vi "Calibrate.vi"(6 "Uncertainty (%) Vin":dbl=1.0, 7 "V_in (V)":dbl=5.0, 8 "Uncertainty (%) Resistor":dbl=1.0, 9 "Resistor (ohms)":dbl=10000.0, 10 "Uncertainty (%) Temp":dbl=1.0, 11 "Temperature (K)":dbl=292.15) -> (0 "Calib Temperature":dbl=292.15, 1 "Uncertainty Calib Temp":dbl=1.0, 2 "Uncertainty (%) Thermistor":dbl=2.9457081958270703, 3 "Calibration Resistance (ohms)":dbl=8620.698071334564, 4 "Canceled":bool, 5 "error out":errorcluster)   [LabVIEW 2013]
panel:
  out "V_out (V)":dbl=2.3148160284617916
  in  "Stop Button":bool
  in  "Calibrate":bool
  in  "Set V_in":bool
  in  "Set V_out":bool
  in  "Set Resistor":bool
  in  "Uncertainty (%) Vout":dbl=1.0
  # "NOTE:\nDO NOT PLAY WITH THIS UNLESS YOU KNOW\nWHAT YOU ARE DOING.\nIncorrect calibration may lead to hardware damage!"
  # "Options"
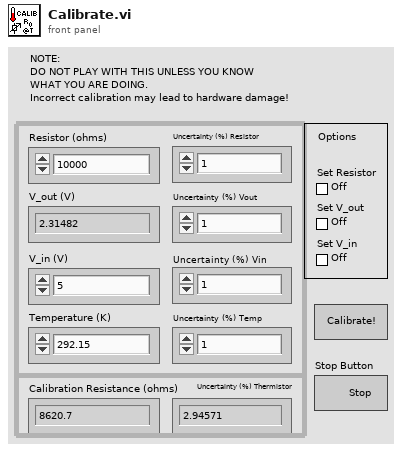
[diagram p1: front panel]
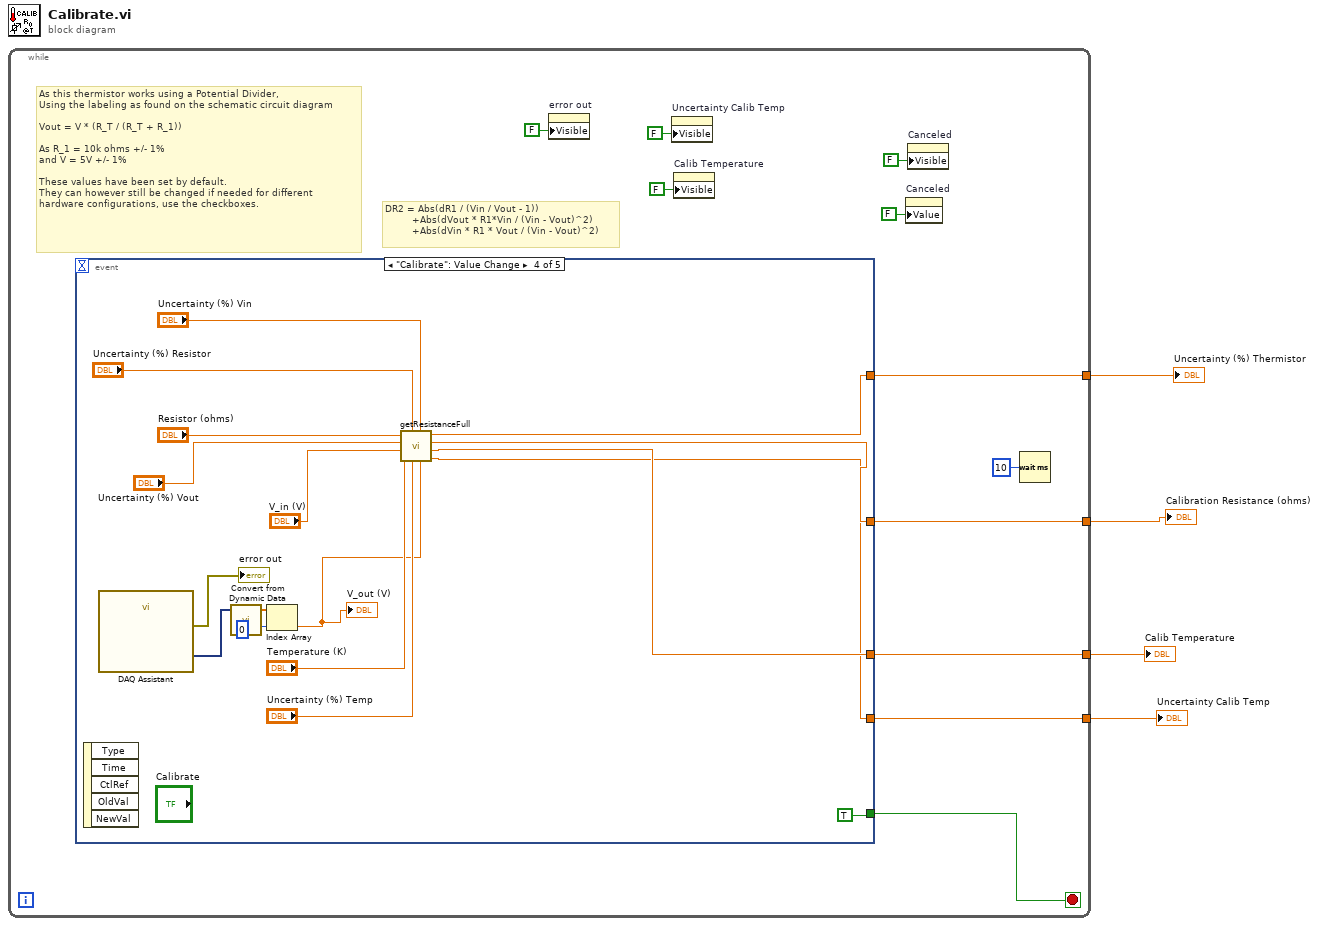
[diagram p0: block diagram]
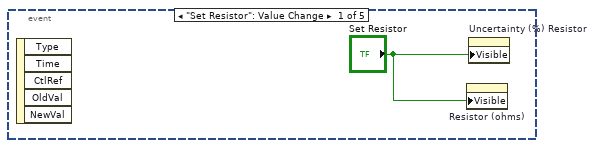
[diagram p2: hidden frame]
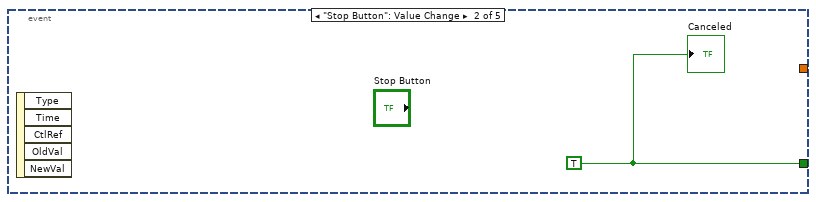
[diagram p3: hidden frame]
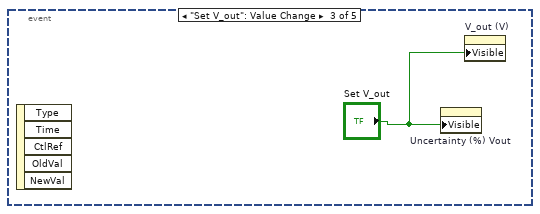
[diagram p4: hidden frame]
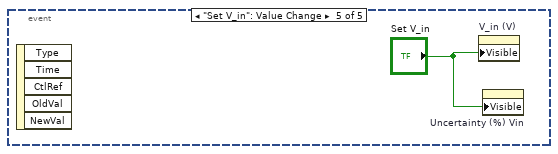
[diagram p5: hidden frame]
diagram:
  n1 = while {
    tunnel: [w9] -> w4
    tunnel: [w8] -> w3
    tunnel: [w7] -> w2
    tunnel: [w6] -> w1
    stop <- w13 stop-if-true
    # "As this thermistor works using a Potential Divider,\nUsing the labeling as found on the schematic circuit diagram\n\nVout = V * (R_T / (R_T + R_1))\n\nAs R_1 = 10k ohms +/- 1%\nand V = 5V +/- 1%\n\nThese values have been set by default.\nThey can however still be changed if needed for different \nhardware configurations, use the checkboxes."
    # "DR2 = Abs(dR1 / (Vin / Vout - 1))\n         +Abs(dVout * R1*Vin / (Vin - Vout)^2)\n         +Abs(dVin * R1 * Vout / (Vin - Vout)^2)"
    n2 = event shown="[3] \"Calibrate\": Value Change" {
      selector: _ -> [_ _ _ _ _]
      dyn-events: _ -> [_ _ _ _ _]
      timeout: _ -> [_ _ _ _ _]
      tunnel: [_ w17 _ TRUE _] -> w13
      tunnel: [_ _ _ w29 _] -> w9
      tunnel: [_ _ _ w28 _] -> w8
      tunnel: [_ _ _ w27 _] -> w7
      tunnel: [_ _ _ w26 _] -> w6
      event "Set Resistor": Value Change {
        n3 = event-data() -> ()  [unwired: 1 in, 5 out]
        n4 = property on="Resistor (ohms)" class="DigNum (strict)"("Visible"="Set Resistor") -> ()  [unwired: 2 in, 2 out]
        n5 = property on="Uncertainty (%) Resistor" class="DigNum (strict)"("Visible"="Set Resistor") -> ()  [unwired: 2 in, 2 out]
      }
      event "Stop Button": Value Change {
        w17 = TRUE
        n6 = event-data() -> ()  [unwired: 1 in, 5 out]
        "Canceled" <- w17
      }
      event "Set V_out": Value Change {
        n7 = event-data() -> ()  [unwired: 1 in, 5 out]
        n8 = property on="Uncertainty (%) Vout" class="DigNum (strict)"("Visible"="Set V_out") -> ()  [unwired: 2 in, 2 out]
        n9 = property on="V_out (V)" class="DigNum (strict)"("Visible"="Set V_out") -> ()  [unwired: 2 in, 2 out]
      }
      event "Calibrate": Value Change {
        n10 = event-data() -> ()  [unwired: 1 in, 5 out]
        n11 = call "DAQ Assistant"() -> ("data"=w19:dynamicdata, "error out"=→"error out":errorcluster)  [unwired: 17 in, 1 out]
        n12 = call "Convert from Dynamic Data"("Dynamic Data Type"=w19) -> ("Array"=w23:dbl[])  [unwired: 3 in]
        n13 = Index Array(array=w23, index=0) -> (element=w21:dbl)
        "V_out (V)" <- w21
        n14 = call "getResistanceFull.vi"("V_out (V)"=w21, "Uncertainty (%) Vin"="Uncertainty (%) Vin", "Uncertainty (%) Temp in"="Uncertainty (%) Temp", "Uncertainty (%) Resistor"="Uncertainty (%) Resistor", "Temperature (K) in"="Temperature (K)", "V_in (V)"="V_in (V)", "Uncertainty (%) Vout"="Uncertainty (%) Vout", "Resistor (ohms)"="Resistor (ohms)") -> ("Uncertainty (%) Temp out"=w26:dbl, "Temperature (K) out"=w27:dbl, "Resistance"=w28:dbl, "Uncertainty"=w29:dbl)
      }
      event "Set V_in": Value Change {
        n15 = event-data() -> ()  [unwired: 1 in, 5 out]
        n16 = property on="V_in (V)" class="DigNum (strict)"("Visible"="Set V_in") -> ()  [unwired: 2 in, 2 out]
        n17 = property on="Uncertainty (%) Vin" class="DigNum (strict)"("Visible"="Set V_in") -> ()  [unwired: 2 in, 2 out]
      }
    }
    n18 = property on="error out" class="Clust (strict)"("Visible"=FALSE) -> ()  [unwired: 2 in, 2 out]
    n19 = property on="Uncertainty Calib Temp" class="DigNum (strict)"("Visible"=FALSE) -> ()  [unwired: 2 in, 2 out]
    n20 = property on="Calib Temperature" class="DigNum (strict)"("Visible"=FALSE) -> ()  [unwired: 2 in, 2 out]
    n21 = property on="Canceled" class="Bool (strict)"("Value"=FALSE ("Canceled")) -> ()  [unwired: 2 in, 2 out]
    n22 = property on="Canceled" class="Bool (strict)"("Visible"=FALSE) -> ()  [unwired: 2 in, 2 out]
    n23 = Wait (ms)(milliseconds to wait=u32 10) -> ()  [unwired: 1 out]
  }
  "Uncertainty (%) Thermistor" <- w4
  "Calibration Resistance (ohms)" <- w3
  "Calib Temperature" <- w2
  "Uncertainty Calib Temp" <- w1
